vi "Pre Launch Init.vi"(11 "SAS_AFTester_Template in":refnum<class "User Interface Tester.lvclass">) -> (0 "error out":errorcluster, 3 "SAS_AFTester_Template out":refnum<class "User Interface Tester.lvclass">)   [LabVIEW 2020, in "User Interface Tester.lvlib" / "User Interface Tester.lvclass"]
doc: "(<B>Filename</B>: Actor Framework.lvlib:Actor.lvclass:Pre Launch Init.vi)\n\nDefines behavior that occurs after the Launch Nested Actor method is invoked but before the actor's Actor Core method begins running.\n\nBy default, this method does nothing. A descendant class may override it to define behavior."
uses:
  User Interface Tester.lvclass
  <vilib>/SAS/Actor Tester/Enqueuer Manager/SAS_AFTester_Enqueuer Manager.lvclass
  User Interface Tester.lvclass/User Interface Tester.ctl
  <vilib>/ActorFramework/Actor/Actor.lvclass
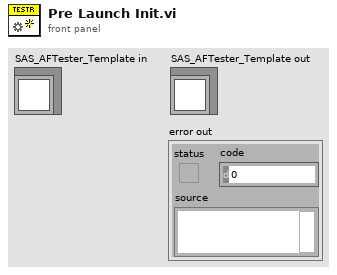
[diagram p1: front panel]
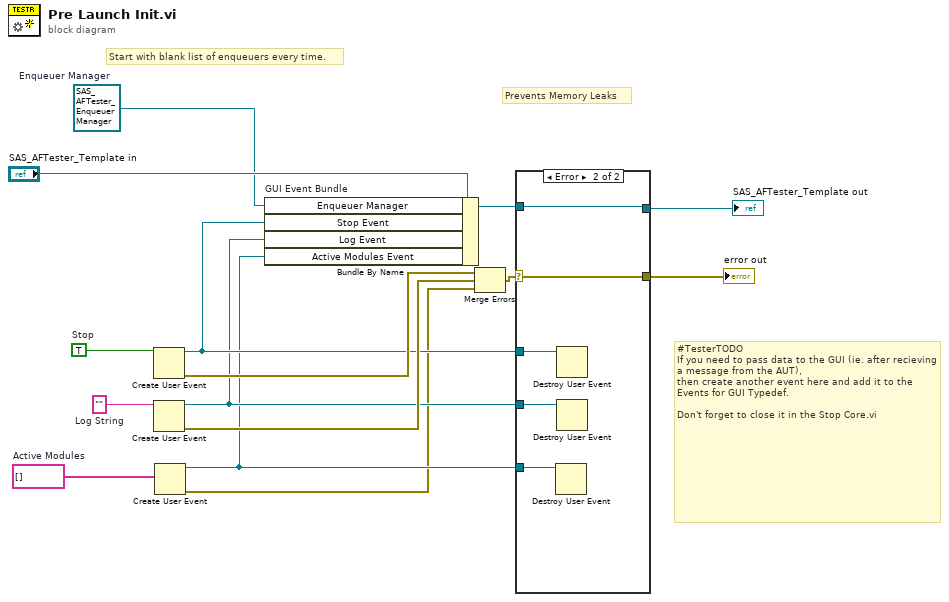
[diagram p0: block diagram]
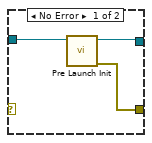
[diagram p2: hidden frame]
diagram:
  w1 = refnum<class "SAS_AFTester_Enqueuer Manager.lvclass"> refnum  # Enqueuer Manager
  w4 = string[] []  # Active Modules
  w11 = TRUE  # Stop
  w12 = ""  # Log String
  # "#TesterTODO\nIf you need to pass data to the GUI (ie. after recieving a message from the AUT),\nthen create another event here and add it to the\nEvents for GUI Typedef.\n\nDon't forget to close it in the Stop Core.vi"
  # "Start with blank list of enqueuers every time."
  # "Prevents Memory Leaks"
  n1 = Create User Event(user event datatype=w11) -> (user event=w6:refnum<user-event>, error out=w9:errorcluster)  [unwired: 1 in]
  n2 = Create User Event(user event datatype=w12) -> (user event=w5:refnum<user-event>, error out=w8:errorcluster)  [unwired: 1 in]
  n3 = Create User Event(user event datatype=w4) -> (user event=w3:refnum<user-event>, error out=w2:errorcluster)  [unwired: 1 in]
  n4 = Bundle By Name "GUI Event Bundle"(cluster="SAS_AFTester_Template in", "Enqueuer Manager"=w1, "Stop Event"=w6, "Log Event"=w5, "Active Modules Event"=w3) -> (w10:refnum<class "User Interface Tester.lvclass">)
  n5 = Merge Errors(w9, w8, w2) -> (w7:errorcluster)
  n6 = case shown="Error" w7 {
    selector: w7 -> [_ w23]
    tunnel: [w18 w23] -> w15
    tunnel: [w17 w22] -> w14
    tunnel: w10 -> [w16 w22]
    tunnel: w6 -> [_ w21]
    tunnel: w5 -> [_ w20]
    tunnel: w3 -> [_ w19]
    frame No Error {
      n7 = call-parent "Pre Launch Init.vi"("Actor in"=w16) -> ("error out"=w18:errorcluster, "Actor out"=w17:refnum<class "User Interface Tester.lvclass">)  [unwired: 9 in]
    }
    frame Error {
      n8 = Destroy User Event(user event=w19) -> ()  [unwired: 1 in, 1 out]
      n9 = Destroy User Event(user event=w21) -> ()  [unwired: 1 in, 1 out]
      n10 = Destroy User Event(user event=w20) -> ()  [unwired: 1 in, 1 out]
    }
  }
  "error out" <- w15
  "SAS_AFTester_Template out" <- w14
